vi "WallAngleFind.vi"(9 "End Angle":i32, 11 "Start Angle":i32) -> (1 "Angle out":dbl, 2 "Y out":dbl, 3 "X out":dbl, 4 "Right Side":dbl, 5 "Left Side":dbl, 6 "Right Point":dbl, 7 "Left Point":dbl)   [LabVIEW 2018]
uses:
  <vilib>/Analysis/coordinate.llb/2D Cartesian Coordinate Rotation (Array).vi
  <vilib>/Analysis/NI_AALPro.lvlib
panel:
  out "Array":dbl[][](array[numeric])
  out "subarray":dbl[](array[numeric])
  out "max index(es)":i32
  out "max value":i32
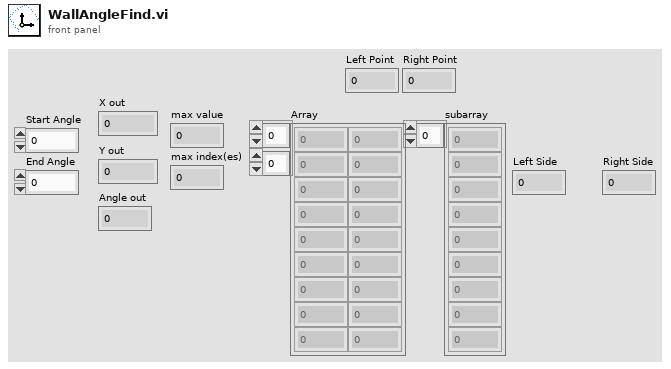
[diagram p1: front panel]
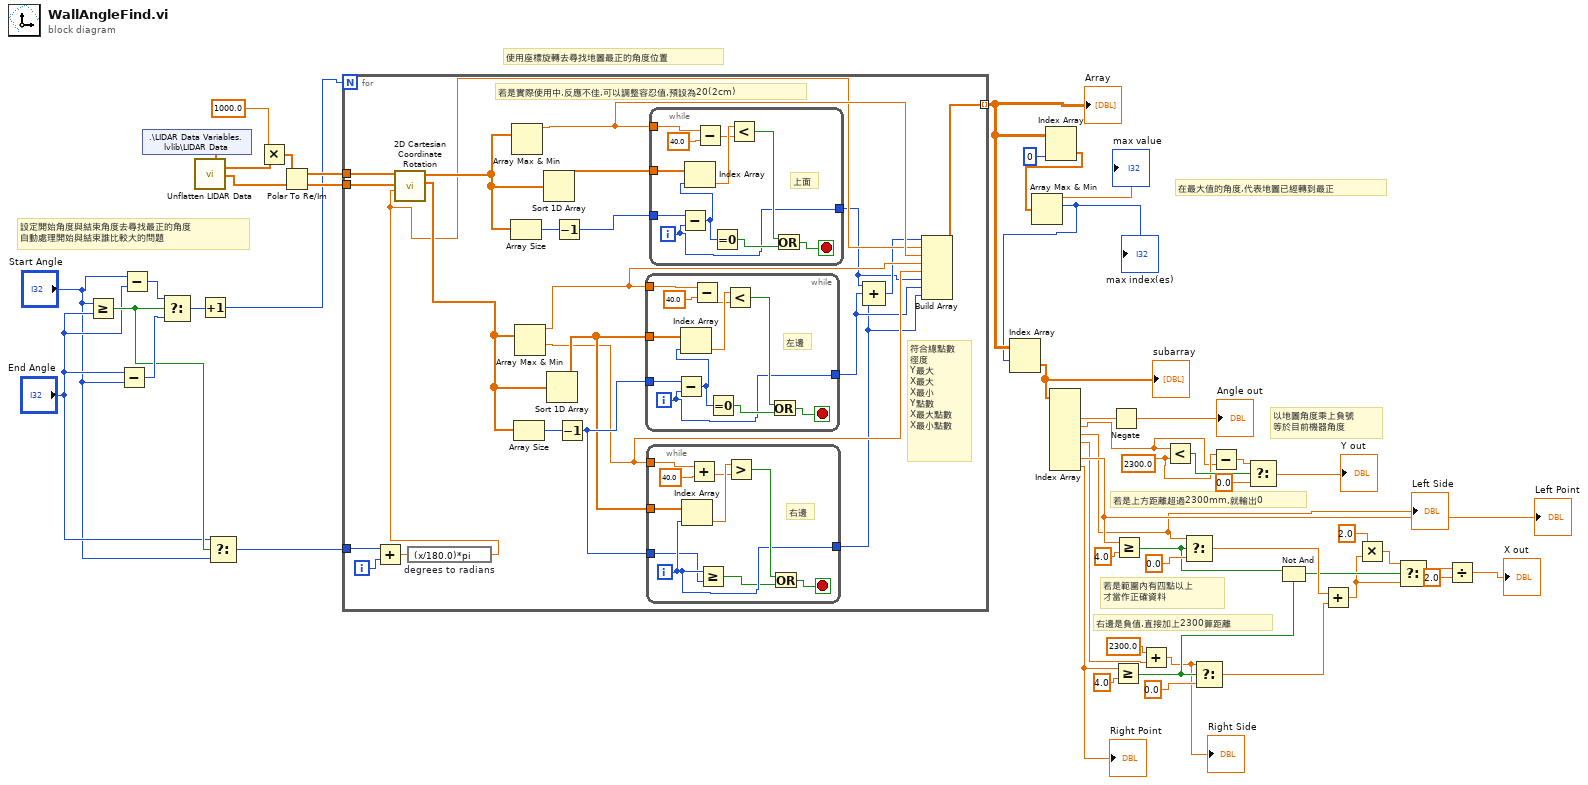
[diagram p0: block diagram]
diagram:
  w26 = 2300.0
  # "右邊是負值,直接加上2300算距離"
  # "若是範圍內有四點以上\n才當作正確資料"
  # "設定開始角度與結束角度去尋找最正的角度\n自動處理開始與結束誰比較大的問題"
  # "使用座標旋轉去尋找地圖最正的角度位置"
  # "在最大值的角度,代表地圖已經轉到最正"
  # "以地圖角度乘上負號\n等於目前機器角度"
  # "若是上方距離超過2300mm,就輸出0"
  n1 = Greater Or Equal?(x="Start Angle", y="End Angle") -> (x >= y?=w32:bool)
  n2 = Subtract(x="End Angle", y="Start Angle") -> (x-y=w35:i32)
  n3 = Subtract(x="Start Angle", y="End Angle") -> (x-y=w36:i32)
  n4 = shared-variable ".\\LIDAR Data Variables.lvlib\\LIDAR Data"() -> (w46:dbl[])  [unwired: 1 in, 1 out]
  n5 = Select(t=w36, s=w32, f=w35) -> (s? t:f=w34:i32)
  n6 = call "Unflatten LIDAR Data.vi"("Flat LIDAR Data"=w46) -> ("Bearing (rad)"=w50:dbl[], "Range (m)"=w47:dbl[])  [unwired: 7 in, 2 out]
  n7 = Increment(x=w34) -> (x+1=w33:i32)
  n8 = Select(t="End Angle", s=w32, f="Start Angle") -> (s? t:f=w29:i32)
  n9 = Multiply(x=1000.0, y=w47) -> (x*y=w49:dbl[])
  n10 = Polar To Re/Im(2:w50, 3:w49) -> (0:w44:dbl[], 1:w45:dbl[])
  n11 = for {
    N: w33 -> [_]
    tunnel: w45 -> [w66]
    tunnel: w44 -> [w65]
    tunnel: [w64] -> w40 mode=indexing
    tunnel: w29 -> [w54]
    i -> [w58]
    # "符合總點數\n徑度\nY最大\nX最大\nX最小\nY點數\nX最大點數\nX最小點數"
    # "若是實際使用中,反應不佳,可以調整容忍值,預設為20(2cm)"
    n12 = Add(x=w54, y=w58) -> (x+y=w57:dbl)
    n13 = expression code="(x/180.0)*pi" "degrees to radians"(w57) -> (w56:dbl)
    n14 = call-poly <vilib>:"2D Cartesian Coordinate Rotation.vi"("theta"=w56, "Y"=w65, "X"=w66) -> ("Y Out"=w59:dbl[], "X Out"=w60:dbl[])  [unwired: 6 in, 1 out]
    n15 = Array Size(array=w60) -> (size(s)=w67:i32)
    n16 = Array Max & Min(array=w60) -> (max value=w63:dbl)  [unwired: 3 out]
    n17 = Array Size(array=w59) -> (size(s)=w70:i32)
    n18 = Array Max & Min(array=w59) -> (max value=w62:dbl, min value=w61:dbl)  [unwired: 2 out]
    n19 = Sort 1D Array(array=w60) -> (sorted array=w69:dbl[])
    n20 = Sort 1D Array(array=w59) -> (sorted array=w71:dbl[])
    n21 = Decrement(x=w67) -> (x-1=w68:i32)
    n22 = Decrement(x=w70) -> (x-1=w72:i32)
    n23 = while {
      tunnel: w72 -> [w93]
      tunnel: w71 -> [w92]
      tunnel: w62 -> [w90]
      tunnel: [w83] -> w52
      i -> [w83]
      stop <- w87 stop-if-true
      # "左邊"
      n24 = Subtract(x=w93, y=w83) -> (x-y=w86:i32)
      n25 = Index Array(array=w92, index=w86) -> (element=w89:dbl)
      n26 = Subtract(x=w90, y=40.0) -> (x-y=w88:dbl)
      n27 = Equal To 0?(x=w86) -> (x = 0?=w85:bool)
      n28 = Less?(x=w89, y=w88) -> (x < y?=w84:bool)
      n29 = Or(x=w84, y=w85) -> (x .or. y?=w87:bool)
    }
    n30 = while {
      tunnel: w72 -> [w74]
      tunnel: w71 -> [w82]
      tunnel: w61 -> [w80]
      tunnel: [w75] -> w51
      i -> [w75]
      stop <- w77 stop-if-true
      # "右邊"
      n31 = Index Array(array=w82, index=w75) -> (element=w79:dbl)
      n32 = Add(x=w80, y=40.0) -> (x+y=w78:dbl)
      n33 = Greater Or Equal?(x=w75, y=w74) -> (x >= y?=w73:bool)
      n34 = Greater?(x=w79, y=w78) -> (0:w76:bool)
      n35 = Or(x=w76, y=w73) -> (x .or. y?=w77:bool)
    }
    n36 = while {
      tunnel: w68 -> [w104]
      tunnel: w69 -> [w103]
      tunnel: w63 -> [w101]
      tunnel: [w94] -> w53
      i -> [w94]
      stop <- w98 stop-if-true
      # "上面"
      n37 = Subtract(x=w104, y=w94) -> (x-y=w97:i32)
      n38 = Index Array(array=w103, index=w97) -> (element=w100:dbl)
      n39 = Subtract(x=w101, y=40.0) -> (x-y=w99:dbl)
      n40 = Equal To 0?(x=w97) -> (x = 0?=w96:bool)
      n41 = Less?(x=w100, y=w99) -> (x < y?=w95:bool)
      n42 = Or(x=w95, y=w96) -> (x .or. y?=w98:bool)
    }
    n43 = Compound Arithmetic op=ADD(w53, w52, w51) -> (w55:i32)
    n44 = Build Array(w55, w56, w63, w62, w61, w53, w52, w51) -> (w64:dbl[])
  }
  "Array" <- w40
  n45 = Index Array(array=w40, index (col)=0 ("disabled index (col)")) -> (element=w42:dbl[])  [unwired: 1 in]
  n46 = Array Max & Min(array=w42) -> (max value=→"max value":dbl, max index (indices)=w39:i32)  [unwired: 2 out]
  "max index(es)" <- w39
  n47 = Index Array(array=w40, index (row)=w39) -> (element=w38:dbl[])  [unwired: 1 in]
  "subarray" <- w38
  n48 = Index Array(array=w38) -> (element #2=w28:dbl, element #3=w25:dbl, element #4=w3:dbl, element #5=w15:dbl, element #7=w22:dbl, element #8=w17:dbl)  [unwired: 8 in, 2 out]
  "Left Side" <- w3
  "Left Point" <- w22
  "Right Point" <- w17
  n49 = Negate(x=w28) -> (-x=→"Angle out":dbl)
  n50 = Greater Or Equal?(x=w17, y=4.0) -> (x >= y?=w13:bool)
  n51 = Greater Or Equal?(x=w22, y=4.0) -> (x >= y?=w14:bool)
  n52 = Add(x=2300.0, y=w15) -> (x+y=w4:dbl)
  "Right Side" <- w4
  n53 = Less?(x=w25, y=w26) -> (x < y?=w27:bool)
  n54 = Select(t=w3, s=w14, f=0.0) -> (s? t:f=w12:dbl)
  n55 = Select(t=w4, s=w13, f=0.0) -> (s? t:f=w11:dbl)
  n56 = Subtract(x=w26, y=w25) -> (x-y=w24:dbl)
  n57 = Select(t=w24, s=w27, f=0.0) -> (s? t:f=→"Y out":dbl)
  n58 = Not And(1:w13, 2:w14) -> (0:w10:bool)
  n59 = Add(x=w12, y=w11) -> (x+y=w5:dbl)
  n60 = Multiply(x=2.0 ("y"), y=w5) -> (x*y=w7:dbl)
  n61 = Select(t=w7, s=w10, f=w5) -> (s? t:f=w9:dbl)
  n62 = Divide(x=w9, y=2.0) -> (x/y=→"X out":dbl)
